vi "Get Connection String.vi"(4 "Error In":errorcluster, 7 "Config Data_DB in":refnum<class "Config Data_DB.lvclass">) -> (0 "Error Out":errorcluster, 2 "Connection String":string, 3 "Config Data_DB out":refnum<class "Config Data_DB.lvclass">)   [LabVIEW 2014, in "Config Data.lvlib" / "Config Data_DB.lvclass"]
uses:
  Config Data_DB.lvclass
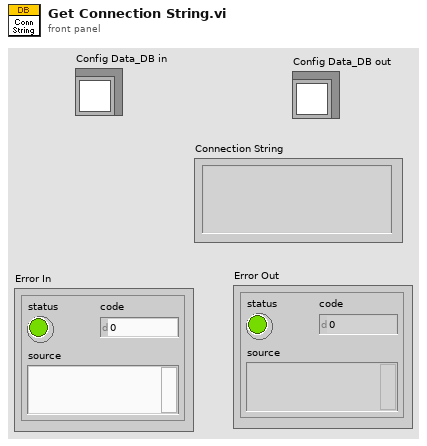
[diagram p1: front panel]
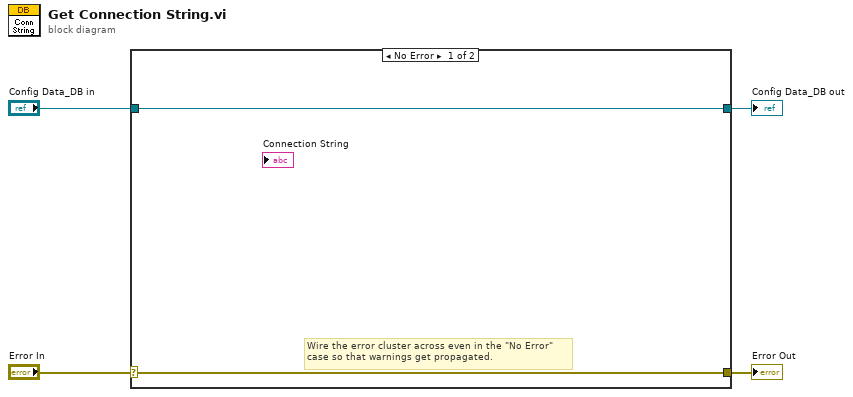
[diagram p0: block diagram]
diagram:
  n1 = case shown="No Error" "Error In" {
    selector: "Error In" -> [w5 w8]
    tunnel: [w5 w8] -> w3
    tunnel: [w6 w7] -> w1
    tunnel: "Config Data_DB in" -> [w6 w7]
    frame No Error {
      # "Wire the error cluster across even in the \"No Error\"\ncase so that warnings get propagated."
    }
    frame Error {
    }
  }
  "Error Out" <- w3
  "Config Data_DB out" <- w1
